vi "addsecuencelocal.vi"() -> ()   [LabVIEW 2020]
panel:
  out "Thermometer":dbl(slide) scale=0.0..100.0
  out "String 2":string
  in  "String":string
  out "Boolean 2":bool
  in  "Boolean":bool
  in  "Numeric":dbl
  # "add secuence local"
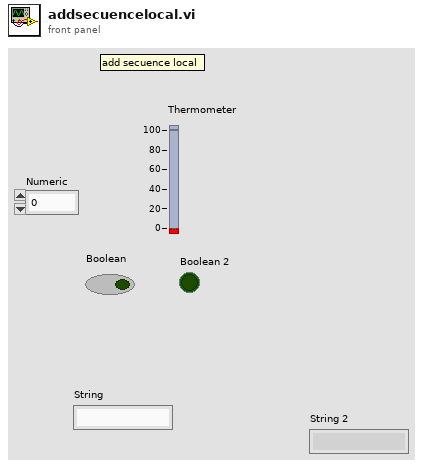
[diagram p1: front panel]
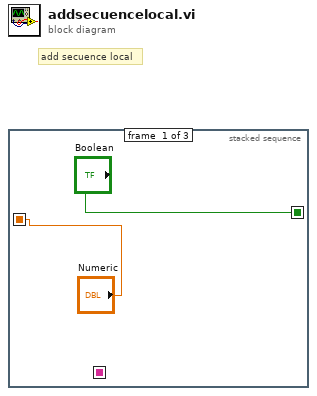
[diagram p0: block diagram]
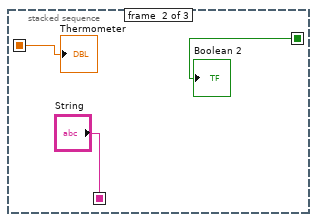
[diagram p2: hidden frame]
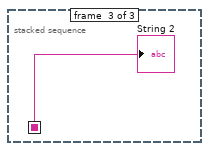
[diagram p3: hidden frame]
diagram:
  # "add secuence local"
  n1 = stacked-sequence {
    seq-local: ["Boolean" _ _] -> [_ w5 _]
    seq-local: ["Numeric" _ _] -> [_ w3 _]
    seq-local: [_ "String" _] -> [_ _ w6]
    frame #0 {
    }
    frame #1 {
      "Boolean 2" <- w5
      "Thermometer" <- w3
    }
    frame #2 {
      "String 2" <- w6
    }
  }
